vi "SH_saveTransform.vi"(7 "Shapelets File":path, 8 "CLassLabels out":string[](array[string]), 9 "Array of Shapelets":cluster{dbl[][]}[](array[cluster]), 10 "ArrayOfTrials":T1(array[cluster]), 11 "Data File":path) -> (0 "error out":errorcluster)   [LabVIEW 2016, in "Shapelets Search (Brute Force).lvlib"]
uses:
  Shapelets Search (Brute Force).lvlib
  _XML_EEG_Features/XML_FF_Header.ctl
  _XML_EEG_Features/XML_FF_Trial.ctl
  <vilib>/Analysis/baseanly.llb/Normalize.vi
  <vilib>/Analysis/baseanly.llb/Normalize Vector.vi
  <vilib>/xml/Close Reference(Node).vi
  _XML_EEG_Features/XML_EEG_Features.lvlib
  <vilib>/xml/NI_XML.lvlib
panel:
  # "This VI is a part of BCI Design library, http://www.ru-bci.org \nCopyright © 2020, Sotnikov Peter, All rights reserved. License: GNU GPLv3"
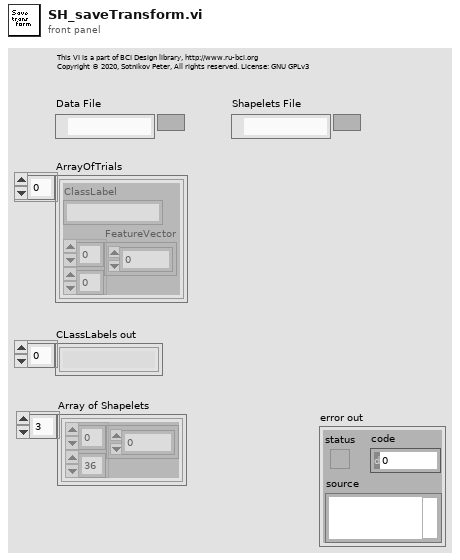
[diagram p1: front panel]
types:
  T1 = cluster{"ClassLabel":string, "FeatureVector":dbl[][]}[]
  T2 = typedef "XML_EEG_Features.lvlib/XML_FF_Trial.ctl" = cluster{"ClassLabel":string, "FeatureVector":dbl[]}
  T3 = typedef "XML_EEG_Features.lvlib/XML_FF_Header.ctl" = cluster{"NumberOfTrials":i32, "NumberOfClasses":i32, "FeatureVectorLength":i32, "FeatureExtractionMethod":string}
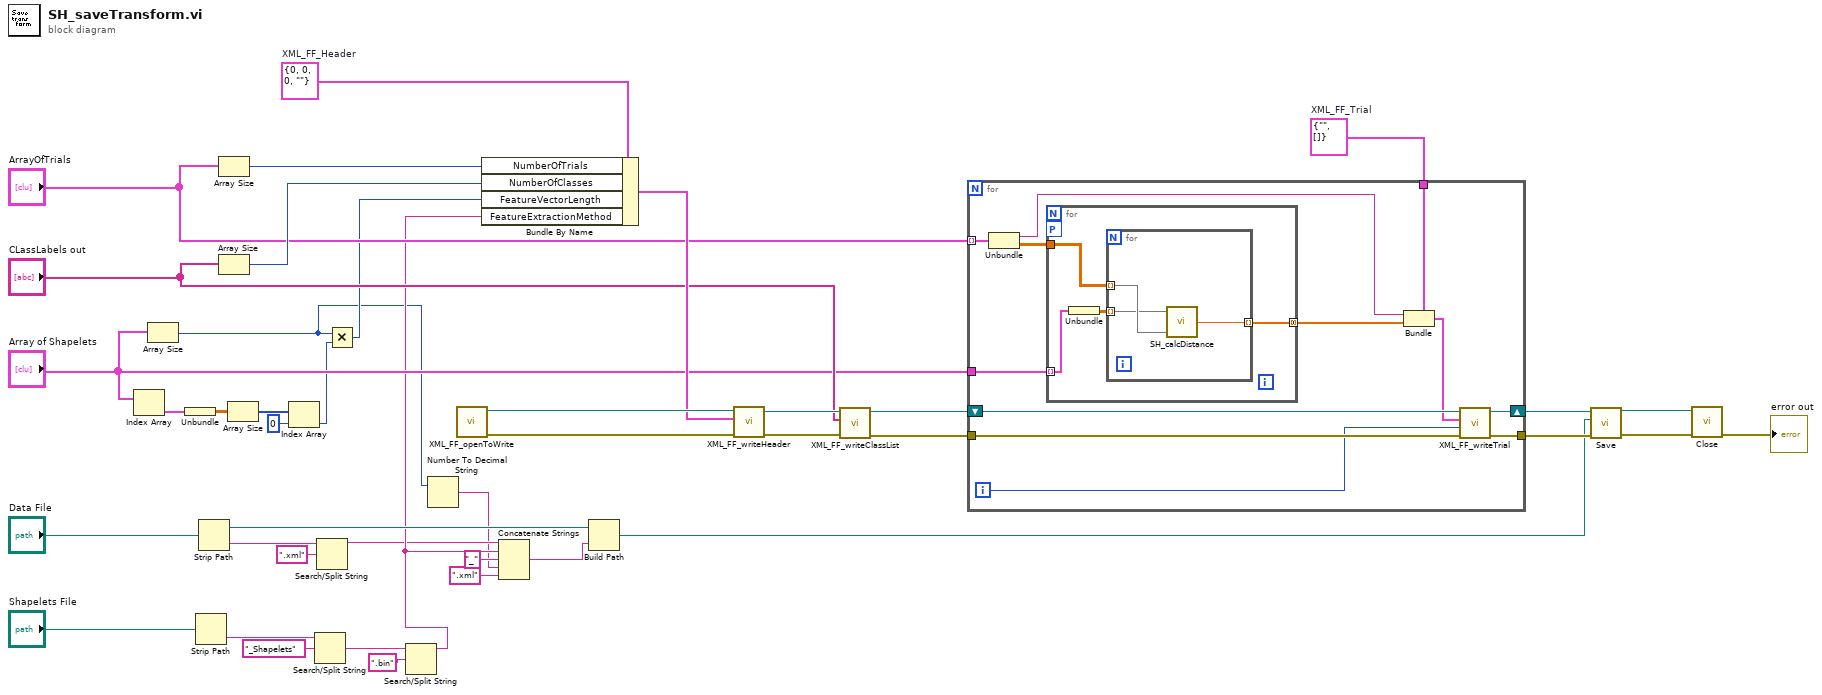
[diagram p0: block diagram]
diagram:
  w24 = T2 {"ClassLabel"="", "FeatureVector"=[]}  # XML_FF_Trial
  w36 = T3 {"NumberOfTrials"=0, "NumberOfClasses"=0, "FeatureVectorLength"=0, "FeatureExtractionMethod"=""}  # XML_FF_Header
  n1 = Index Array(array="Array of Shapelets") -> (element=w16:cluster{dbl[][]})  [unwired: 1 in]
  n2 = Array Size(array="Array of Shapelets") -> (size(s)=w3:i32)
  n3 = Unbundle(w16) -> (w15:dbl[][])
  n4 = Strip Path(path="Shapelets File") -> (name=w11:string)  [unwired: 1 out]
  n5 = Strip Path(path="Data File") -> (stripped path=w38:path, name=w41:string)
  n6 = Array Size(array="ArrayOfTrials") -> (size(s)=w35:i32)
  n7 = Array Size(array="CLassLabels out") -> (size(s)=w34:i32)
  n8 = Array Size(array=w15) -> (size(s)=w14:i32[])
  n9 = Index Array(array=w14, index=0) -> (element=w5:i32)
  n10 = Search/Split String(string=w11, search string/char (-)="_Shapelets") -> (match + rest of string=w8:string)  [unwired: 1 in, 2 out]
  n11 = Search/Split String(string=w41, search string/char (-)=".xml") -> (substring before match=w6:string)  [unwired: 1 in, 2 out]
  n12 = Multiply(x=w3, y=w5) -> (x*y=w4:i32)
  n13 = Search/Split String(string=w8, search string/char (-)=".bin") -> (substring before match=w7:string)  [unwired: 1 in, 2 out]
  n14 = Number To Decimal String(number=w3) -> (decimal integer string=w2:string)  [unwired: 1 in]
  n15 = call "XML_FF_openToWrite.vi"() -> ("error out"=w32:errorcluster, "DOM document out"=w33:refnum<k20>)  [unwired: 10 in]
  n16 = Bundle By Name(cluster=w36, "NumberOfTrials"=w35, "NumberOfClasses"=w34, "FeatureVectorLength"=w4, "FeatureExtractionMethod"=w7) -> (w31:T3)
  n17 = Concatenate Strings(w6, w7, "_" ("string"), w2, ".xml" ("string")) -> (w37:string)
  n18 = Build Path(base path=w38, name or relative path=w37) -> (appended path=w21:path)
  n19 = call "XML_FF_writeHeader.vi"("error in (no error)"=w32, "XML_FF_Header"=w31, "DOM document in"=w33) -> ("error out"=w30:errorcluster, "DOM document out"=w29:refnum<k20>)  [unwired: 7 in]
  n20 = call "XML_FF_writeClassList.vi"("error in (no error)"=w30, "ClassList"="CLassLabels out", "DOM document in"=w29) -> ("error out"=w27:errorcluster, "DOM document out"=w26:refnum<k20>)  [unwired: 7 in]
  n21 = for {
    tunnel: w27 -> [w53]
    shift-right: [w51] -> w22
    shift-left: w26 -> [w54]
    tunnel: "ArrayOfTrials" -> [w50] mode=indexing
    tunnel: "Array of Shapelets" -> [w49]
    tunnel: w24 -> [w45]
    tunnel: [w44] -> w23
    i -> [w52]
    n22 = Unbundle(w50) -> ("ClassLabel"=w47:string, "FeatureVector"=w48:dbl[][])
    n23 = for {
      tunnel: w49 -> [w56] mode=indexing
      tunnel: w48 -> [w58]
      tunnel: [w57] -> w43 mode=concatenating
      workers-P: _ -> [_]
      n24 = Unbundle(w56) -> (w55:dbl[][])
      n25 = for {
        tunnel: w58 -> [w61] mode=indexing
        tunnel: [w60] -> w57 mode=indexing
        tunnel: w55 -> [w59] mode=indexing
        n26 = call "SH_calcDistance.vi"("Time series"=w61, "Shapelet (normalized)"=w59) -> ("Distance out"=w60:dbl)  [unwired: 1 in]
      }
    }
    n27 = Bundle(cluster=w45, "ClassLabel"=w47, "FeatureVector"=w43) -> (w46:T2)
    n28 = call "XML_FF_writeTrial.vi"("error in (no error)"=w53, "Trial Number"=w52, "XML_FF_Trial"=w46, "DOM document in"=w54) -> ("error out"=w44:errorcluster, "DOM document out"=w51:refnum<k20>)  [unwired: 6 in]
  }
  n29 = call <vilib>:"Save.vi"("error in (no error)"=w23, "XML file path"=w21, "DOM document in"=w22) -> ("error out"=w19:errorcluster, "DOM document out"=w20:refnum<k20>)  [unwired: 6 in, 1 out]
  n30 = call-poly <vilib>:"Close.vi"("error in (no error)"=w19, "node"=w20) -> ("error out"=→"error out":errorcluster)  [unwired: 7 in]
